vi "Sum_of_Gaussians.vi"(8 "X_array":i32[](array[numeric]), 11 "Y_array":i32[](array[numeric])) -> (0 "Gauss 3 fit":cluster{"a":dbl, "m":dbl, "sigma":dbl}, 1 "Gauss 2 fit":cluster{"a":dbl, "m":dbl, "sigma":dbl}, 2 "Gauss 1 fit":cluster{"a":dbl, "m":dbl, "sigma":dbl}, 3 "best nonlinear fit":dbl[](array[numeric]))   [LabVIEW 2015]
doc: "Demonstrates fitting data to a model that is the sum of three Gaussian curves and an offset."
uses:
  <vilib>/Utility/error.llb/DialogType.ctl
  <vilib>/gmath/NumericalOptimization/Nonlinear Curve Fit LM.vi
  <vilib>/gmath/NI_Gmath.lvlib
  <vilib>/Analysis/NI_AAL_SigProc.lvlib
panel:
  out "Gaussian fit":T1(graph)
  out "Number of function calls":i32
  out "Residue":dbl
  # "Overview: Demonstrates fitting data to a model that is the sum of three Gaussian curves and an offset.\nRequirements: LabVIEW Full Development System\nInstructions:\n1.  Run the VI.\n2.  Notice the fit, which is mostly good.  Sometimes the smallest peak is missed due to the starting set of parameters for the fit.\n3.  Change the Gaussian parameters (DC offset, Gauss 1, Gauss 2, and Gauss 3) or Noise sigma and run the VI again."
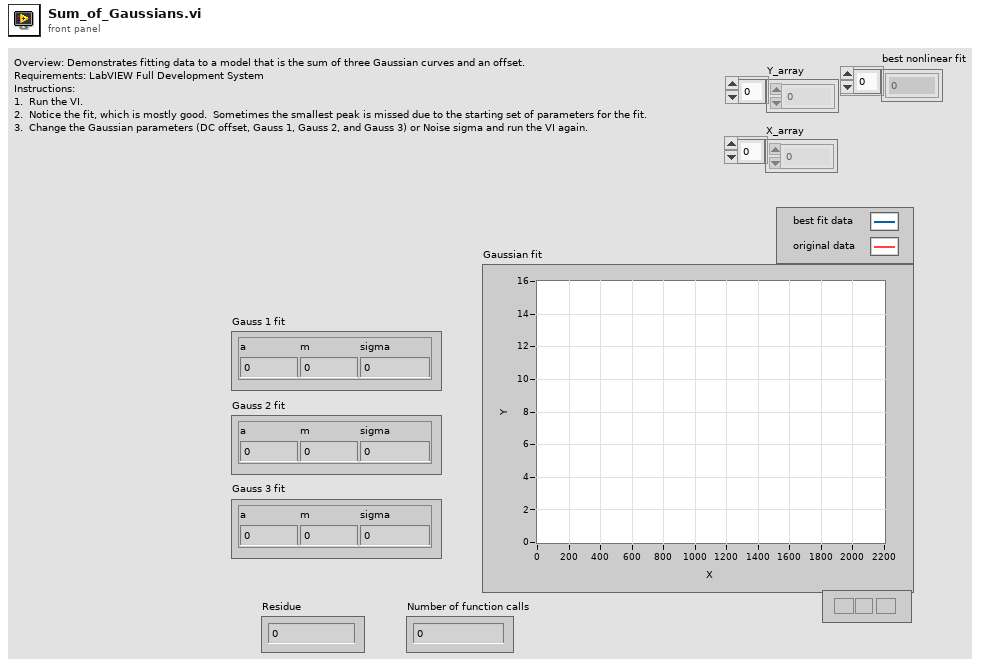
[diagram p1: front panel]
types:
  T1 = cluster{"X_array":i32[], "best nonlinear fit":dbl[]}[]
  T2 = typedef "DialogType.ctl" = u16
  T3 = cluster{"X_array":i32[], "best nonlinear fit":dbl[]}
  T4 = cluster{"Numeric":dbl, "Numeric":dbl, "Numeric":dbl}
  T5 = cluster{"Numeric":dbl, "Numeric":dbl, "Numeric":dbl}[]
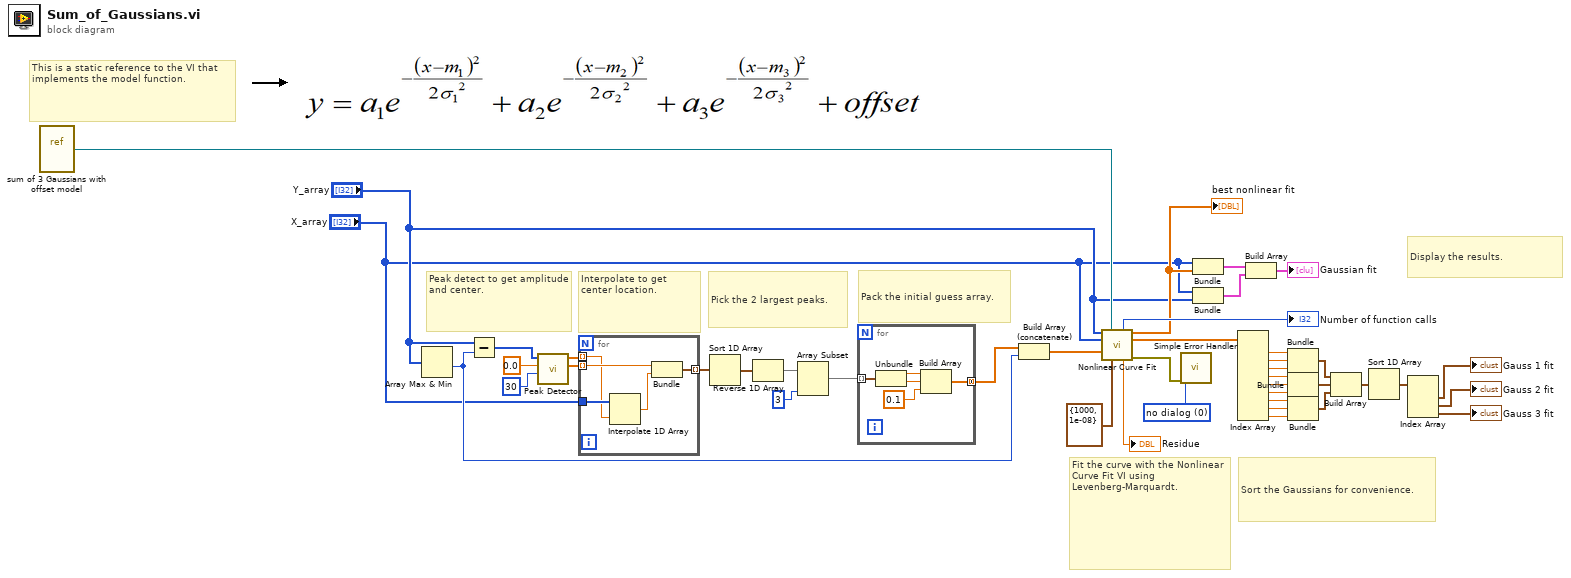
[diagram p0: block diagram]
diagram:
  w1 = T2 0 items=["no dialog", "OK message", "continue or stop message", "OK message + warnings", "continue/stop + warnings"] ("type of dialog (OK msg:1)")
  # "Pack the initial guess array."
  # "Pick the 2 largest peaks."
  # "Peak detect to get amplitude and center."
  # "Sort the Gaussians for convenience."
  # "Display the results."
  # "Fit the curve with the Nonlinear Curve Fit VI using Levenberg-Marquardt."
  # "Interpolate to get center location."
  # "This is a static reference to the VI that implements the model function."
  n1 = vi-ref "sum of 3 Gaussians with offset model.vi"() -> (w5:refnum<vi>)
  n2 = Array Max & Min(array="Y_array") -> (min value=w8:i32)  [unwired: 3 out]
  n3 = Subtract(x="Y_array", y=w8) -> (x-y=w14:i32[])
  n4 = call <vilib>:"Peak Detector.vi"("width"=30, "threshold"=0.0, "X"=w14) -> ("Amplitudes"=w17:dbl[], "Locations"=w16:dbl[])  [unwired: 4 in, 3 out]
  n5 = for {
    tunnel: w17 -> [w48] mode=indexing
    tunnel: w16 -> [w45] mode=indexing
    tunnel: [w47] -> w15 mode=indexing
    tunnel: "X_array" -> [w46]
    n6 = Interpolate 1D Array(1:w45, 2:w46) -> (0:w44:dbl)
    n7 = Bundle(w48, w44) -> (w47:cluster{dbl, dbl})  [unwired: 1 in]
  }
  n8 = Sort 1D Array(array=w15) -> (sorted array=w13:cluster{dbl, dbl}[])
  n9 = Reverse 1D Array(array=w13) -> (reversed array=w12:cluster{dbl, dbl}[])
  n10 = Array Subset(array=w12, length=3) -> (w9:cluster{dbl, dbl}[])  [unwired: 1 in]
  n11 = for {
    tunnel: w9 -> [w53] mode=indexing
    tunnel: [w49] -> w4 mode=concatenating
    n12 = Unbundle(w53) -> (w52:dbl, w51:dbl)
    n13 = Build Array(w52, w51, 0.1) -> (w49:dbl[])
  }
  n14 = Build Array (concatenate)(w4, w8) -> (w7:dbl[])
  n15 = call-poly <vilib>:"Nonlinear Curve Fit.vi"("Y"="Y_array", "f(x,a)"=w5, "X"="X_array", "initial parameters"=w7, "termination"=cluster{"max iteration":i32, "tolerance":dbl} {"max iteration"=1000, "tolerance"=1e-08}) -> ("number of function calls"=→"Number of function calls":i32, "best nonlinear fit"=w42:dbl[], "best fit parameters"=w40:dbl[], "residue"=→"Residue":dbl, "error out"=w6:errorcluster)  [unwired: 5 in, 1 out]
  "best nonlinear fit" <- w42
  n16 = call <vilib>:"Simple Error Handler.vi"("type of dialog (OK msg:1)"=w1, "error in (no error)"=w6) -> ()  [unwired: 3 in, 5 out]
  n17 = Bundle("X_array"="X_array", "best nonlinear fit"=w42) -> (w27:T3)  [unwired: 1 in]
  n18 = Bundle("X_array"="X_array", "Y_array"="Y_array") -> (w28:cluster{"X_array":i32[], "Y_array":i32[]})  [unwired: 1 in]
  n19 = Index Array(array=w40) -> (element #1=w39:dbl, element #2=w38:dbl, element #3=w37:dbl, element #4=w36:dbl, element #5=w35:dbl, element #6=w34:dbl, element #7=w33:dbl, element #8=w32:dbl, element #9=w31:dbl)  [unwired: 9 in]
  n20 = Build Array(w27, w28) -> (→"Gaussian fit":T1)
  n21 = Bundle("Numeric"=w39, "Numeric"=w38, "Numeric"=w37) -> (w26:T4)  [unwired: 1 in]
  n22 = Bundle("Numeric"=w36, "Numeric"=w35, "Numeric"=w34) -> (w25:T4)  [unwired: 1 in]
  n23 = Bundle("Numeric"=w33, "Numeric"=w32, "Numeric"=w31) -> (w24:T4)  [unwired: 1 in]
  n24 = Build Array(w26, w25, w24) -> (w23:T5)
  n25 = Sort 1D Array(array=w23) -> (sorted array=w22:T5)
  n26 = Index Array(array=w22) -> (element #1=→"Gauss 1 fit":T4, element #2=→"Gauss 2 fit":T4, element #3=→"Gauss 3 fit":T4)  [unwired: 3 in]
